vi "GV gated line clock.vi"() -> ()   [LabVIEW 2017]
panel:
  out "Gated line clock":bool
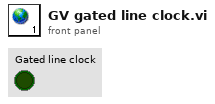
[diagram p1: front panel]
diagram:
